vi "New SpreadsheetDocument.vi"(7 "ooCalc":refnum<class "ooCalc.lvclass">, 8 "error in (no error)":errorcluster, 10 "template (empty)":path) -> (0 "error out":errorcluster, 3 "ooCalc out":refnum<class "ooCalc.lvclass">)   [LabVIEW 2009, in "ooCalc.lvclass"]
uses:
  ooCalc.lvclass
  C:/Projets/LAVAG/OpenOfficeRGT/AODL/DLLs/AODL.dll
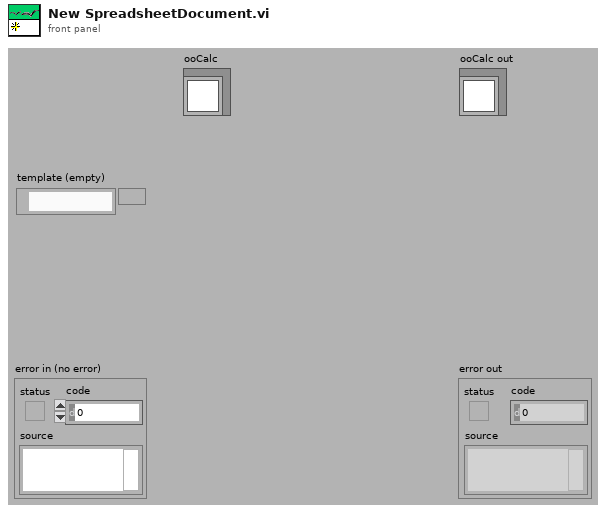
[diagram p1: front panel]
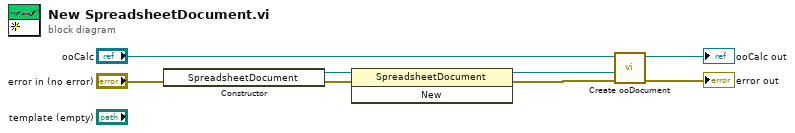
[diagram p0: block diagram]
diagram:
  n1 = constructor class="SpreadsheetDocument"(error in="error in (no error)") -> (reference out=w8:refnum<k24>, error out=w7:errorcluster)  [unwired: 2 in, 1 out]
  n2 = invoke class="SpreadsheetDocument" method="New"(reference=w8, error in=w7) -> (reference out=w1:refnum<k24>, error out=w3:errorcluster)  [unwired: 1 in, 1 out]
  n3 = call-dynamic "Create ooDocument.vi"("error in (no error)"=w3, "Document"=w1, "ooDocument in"="ooCalc") -> ("error out"=→"error out":errorcluster, "ooDocument out"=→"ooCalc out":refnum<class "ooCalc.lvclass">)  [unwired: 7 in]
